vi "PIM Translate Hardware Errors.vi"(8 "error in (no error)":errorcluster) -> (0 "error out":errorcluster)   [LabVIEW 2011]
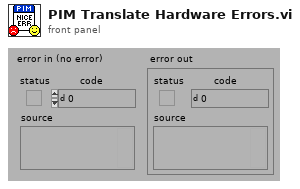
[diagram p1: front panel]
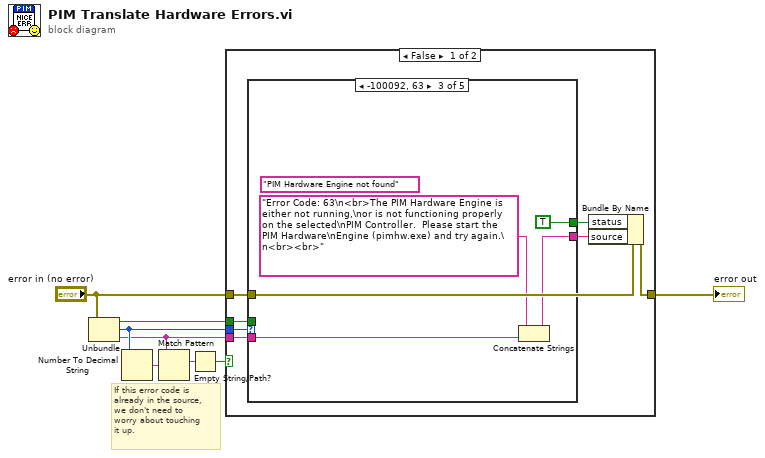
[diagram p0: block diagram]
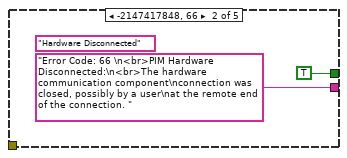
[diagram p3: hidden frame]
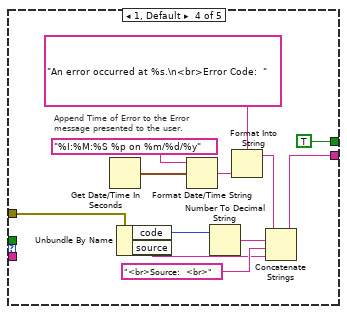
[diagram p4: hidden frame]
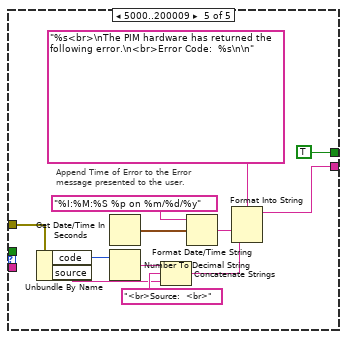
[diagram p5: hidden frame]
diagram:
  # "If this error code is\nalready in the source,\nwe don't need to\nworry about touching\nit up."
  n1 = Unbundle("error in (no error)") -> ("status"=w6:bool, "code"=w5:i32, "source"=w4:string)
  n2 = Number To Decimal String(number=w5) -> (decimal integer string=w3:string)  [unwired: 1 out]
  n3 = Match Pattern(string=w4, regular expression=w3) -> (match substring=w2:string)  [unwired: 4 out]
  n4 = Empty String/Path?(string/path=w2) -> (empty?=w1:bool)
  n5 = case shown="False" w1 {
    tunnel: w4 -> [w15 _]
    tunnel: w5 -> [w14 _]
    tunnel: "error in (no error)" -> [w12 w48]
    tunnel: [w11 w48] -> w7
    tunnel: w6 -> [w9 _]
    frame False {
      n6 = case shown="-100092, 63" w14 {
        tunnel: w12 -> [_ _ _ w33 w45]
        tunnel: w15 -> [w17 _ w21 _ _]
        tunnel: [w17 "Error Code: 66 \n<br>PIM Hardware Disconnected:\n<br>The hardware communication component\nconnection was closed, possibly by a user\nat the remote end of the connection. " w20 w25 w37] -> w13
        tunnel: [w16 TRUE ("status") TRUE ("status") TRUE ("status") TRUE ("status")] -> w10
        tunnel: w9 -> [w16 _ _ _ _]
        frame 0, 200010 {
        }
        frame -2147417848, 66 {
          (unwired) "Hardware Disconnected"
        }
        frame -100092, 63 {
          (unwired) "PIM Hardware Engine not found"
          n7 = Concatenate Strings("Error Code: 63\n<br>The PIM Hardware Engine is either not running,\nor is not functioning properly on the selected\nPIM Controller.  Please start the PIM Hardware\nEngine (pimhw.exe) and try again.\n<br><br>", w21) -> (w20:string)
        }
        frame 1, Default {
          # "Append Time of Error to the Error\nmessage presented to the user."
          n8 = Get Date/Time In Seconds() -> (seconds since 1Jan1904=w29:timestamp)
          n9 = Unbundle By Name(w33) -> ("code"=w32:i32, "source"=w31:string)
          n10 = Format Date/Time String(time format string (%c)="%I:%M:%S %p on %m/%d/%y", seconds (now)=w29) -> (date/time string=w28:string)  [unwired: 1 out]
          n11 = Number To Decimal String(number=w32) -> (decimal integer string=w35:string)  [unwired: 1 out]
          n12 = Format Into String(format string="An error occurred at %s.\n<br>Error Code:  ", w28) -> (resulting string=w26:string)  [unwired: 2 in, 1 out]
          n13 = Concatenate Strings(w26, w35, "<br>Source:  <br>", w31) -> (w25:string)
        }
        frame 5000..200009 {
          # "Append Time of Error to the Error\nmessage presented to the user."
          n14 = Unbundle By Name(w45) -> ("code"=w44:i32, "source"=w43:string)
          n15 = Get Date/Time In Seconds() -> (seconds since 1Jan1904=w41:timestamp)
          n16 = Number To Decimal String(number=w44) -> (decimal integer string=w47:string)  [unwired: 1 out]
          n17 = Concatenate Strings(w47, "<br>Source:  <br>", w43) -> (w38:string)
          n18 = Format Date/Time String(time format string (%c)="%I:%M:%S %p on %m/%d/%y", seconds (now)=w41) -> (date/time string=w40:string)  [unwired: 1 out]
          n19 = Format Into String(format string="%s<br>\nThe PIM hardware has returned the following error.\n<br>Error Code:  %s\n\n", w40, w38) -> (resulting string=w37:string)  [unwired: 2 in, 1 out]
        }
      }
      n20 = Bundle By Name(cluster=w12, "status"=w10, "source"=w13) -> (w11:errorcluster)
    }
    frame True {
    }
  }
  "error out" <- w7
